vi "subVI_QCM.vi"(8 "error in (no error)":errorcluster, 9 "Loop iteration number":i32, 10 "millisecond timer value":u32, 11 "VISA Refnum in":refnum<visa-resource-name>) -> (0 "error out":errorcluster, 1 "Resistance (Ohm)":string, 2 "Freq (Hz)":string, 3 "VISA Refnum out":refnum<visa-resource-name>, 5 "Freq and Resistance Graph":T1(graph))   [LabVIEW 2013]
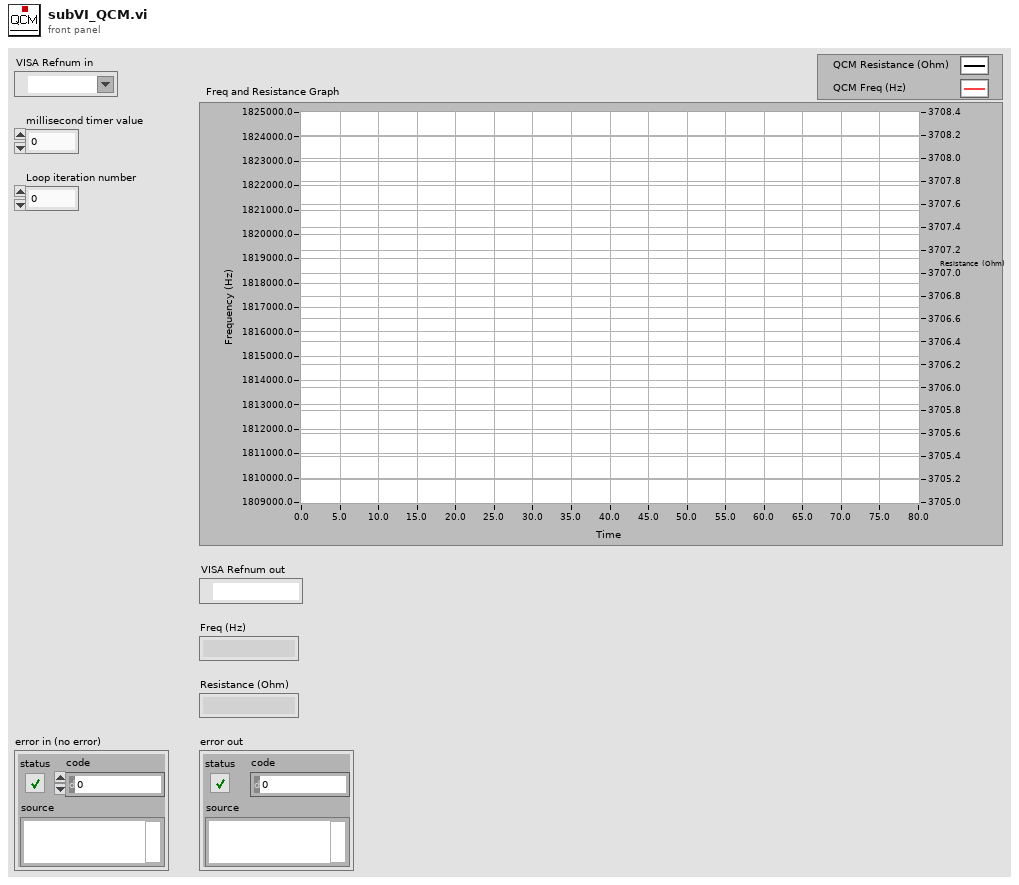
[diagram p1: front panel]
types:
  T1 = cluster{"XY chart data":cluster{"x":dbl, "y":dbl}[]}[]
  T2 = cluster{"timestamp out":dbl, "Frequency out":dbl}
  T3 = cluster{"timestamp out":dbl, "Resistance out":dbl}
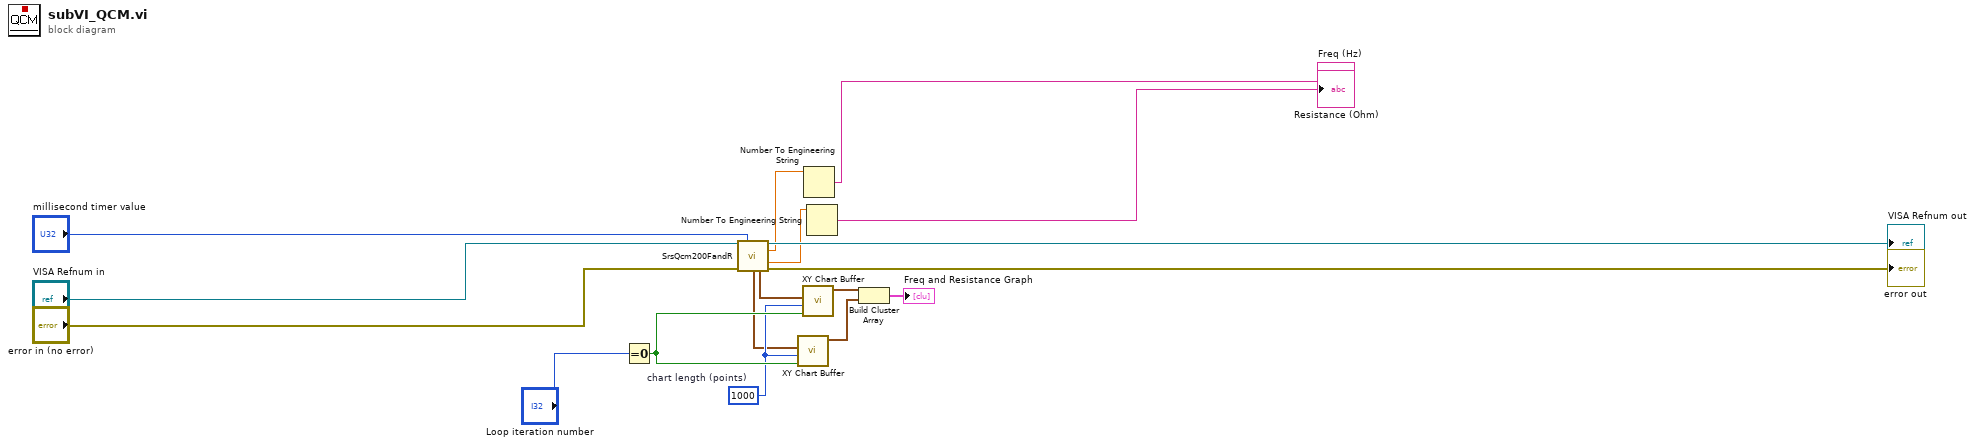
[diagram p0: block diagram]
diagram:
  w3 = 1000  # chart length (points)
  n1 = Equal To 0?(x="Loop iteration number") -> (x = 0?=w7:bool)
  n2 = call <instrlib>:"SrsQcm200FandR.vi"("VISA in"="VISA Refnum in", "Reference time in"="millisecond timer value", "error in (no error)"="error in (no error)") -> ("VISA out"=→"VISA Refnum out":refnum<visa-resource-name>, "Frequency out"=w8:dbl, "Resistance out"=w9:dbl, "F vs T out"=w1:T2, "R vs T out"=w2:T3, "error out"=→"error out":errorcluster)  [unwired: 6 in, 1 out]
  n3 = call <instrlib>:"XY Chart Buffer.vi"("clear first (no:F)"=w7, "chart length (points)"=w3, "new point"=w1) -> ("XY chart data"=w5:cluster{"x":dbl, "y":dbl}[])  [unwired: 8 in]
  n4 = call <instrlib>:"XY Chart Buffer.vi"("clear first (no:F)"=w7, "chart length (points)"=w3, "new point"=w2) -> ("XY chart data"=w4:cluster{"x":dbl, "y":dbl}[])  [unwired: 8 in]
  n5 = Number To Engineering String(4:w8) -> (0:→"Freq (Hz)":string)  [unwired: 3 in]
  n6 = Number To Engineering String(4:w9) -> (0:→"Resistance (Ohm)":string)  [unwired: 3 in]
  n7 = Build Cluster Array(w4, w5) -> (→"Freq and Resistance Graph":T1)
